vi "Measurement Logic.vi"() -> ()   [LabVIEW 2024, in "Averaged - Broadband.lvlib"]
uses:
  Averaged - Broadband.lvlib
  <vilib>/Plug-In SDKs/Measurements/Measure Call Context/Measure Call Context.lvclass
  Measurement Configuration.ctl
  Measurement Results.ctl
  <vilib>/addons/_NISVFA/_Generation/Signal Generation/SV Signal/sv_System Timing Model.ctl
  Program Files/NI/LVAddons/nisvt/1/examples/Sound and Vibration/Audio Measurements/subVIs/sv_AI Channel Configuration.ctl
  Program Files/NI/LVAddons/nisvt/1/examples/Sound and Vibration/Audio Measurements/subVIs/sv_AO Channel Configuration.ctl
  <vilib>/addons/_NISVFA/_Shared subVIs/Controls/NI Spectrum Component.ctl
  <vilib>/addons/_NISVFA/_Shared subVIs/Controls/svc_Window [Dual FFT].ctl
  <vilib>/addons/_NISVFA/_Generation/Signal Generation/SV Signal/SV Signal.lvclass/SV Signal.ctl
  <vilib>/addons/_NISVFA/_Generation/Signal Generation/SV Signal/Write Number of Averages.vi
  <extravilib>/ChannelInstances/High Speed Stream-a[.](wfm(dbl))/_Read For Replicate.vi
  <extravilib>/ChannelInstances/Tag-bool/Write.vi
  <vilib>/DAQmx/read.llb/DAQmx Read.vi
  <vilib>/DAQmx/read.llb/DAQmx Read (Analog 1D Wfm NChan NSamp Duration).vi
  <extravilib>/ChannelInstances/High Speed Stream-a[.](wfm(dbl))/Write.vi
  <vilib>/DAQmx/write.llb/DAQmx Write.vi
  <vilib>/DAQmx/write.llb/DAQmx Write (Analog Wfm 1Chan NSamp).vi
  Program Files/NI/LVAddons/nisvt/1/examples/Sound and Vibration/Audio Measurements/subVIs/sv_Synchronization Gatekeeper.vi
  <vilib>/Utility/error.llb/Clear Errors.vi
  Program Files/NI/LVAddons/nisvt/1/examples/Sound and Vibration/Audio Measurements/subVIs/sv_Align and Parse for Stimulus Response.vi
  Program Files/NI/LVAddons/nisvt/1/examples/Sound and Vibration/Audio Measurements/subVIs/sv_Synchronize Acquisition and Generation.vi
  Program Files/NI/LVAddons/nisvt/1/examples/Sound and Vibration/Audio Measurements/subVIs/sv_Synchronize DSA AI and AO Tasks.vi
  <extravilib>/ChannelInstances/Tag-bool/Read With Abort.vi
  <extravilib>/ChannelInstances/Tag-bool/Write With Abort.vi
  Program Files/NI/LVAddons/nisvt/1/examples/Sound and Vibration/Audio Measurements/subVIs/sv_Prepare Acquired Waveforms for Parsing.vi
  Program Files/NI/LVAddons/nisvt/1/examples/Sound and Vibration/Audio Measurements/subVIs/sv_Timing for Stimulus Response Tasks.vi
  <vilib>/addons/_NISVFA/_Generation/Signal Generation/SV Signal/Read Total Samples.vi
  <vilib>/addons/_NISVFA/_Generation/Signal Generation/SV Signal/Write Leading Synchronization Pulse Enable.vi
  Program Files/NI/LVAddons/nisvt/1/examples/Sound and Vibration/Audio Measurements/subVIs/sv_Synchronization Keymaster.vi
  Program Files/NI/LVAddons/nisvt/1/examples/Sound and Vibration/Audio Measurements/subVIs/sv_Get Reference Clock.vi
  Program Files/NI/LVAddons/nisvt/1/examples/Sound and Vibration/Audio Measurements/subVIs/sv_Synchronization Keymaster_GO.vi
  <extravilib>/ChannelInstances/Tag-c(ref(UserDefinedRefnumTag),t'Rendezvous RefNum')/Read With Abort.vi
  Program Files/NI/LVAddons/nisvt/1/examples/Sound and Vibration/Audio Measurements/subVIs/sv_Align Waveforms by Leading Sync Pulse.vi
  <vilib>/addons/_NISVFA/_Generation/Signal Generation/SV Signal/Read Synchronization Pulse Waveform.vi
  <vilib>/addons/_NISVFA/_Shared subVIs/Common/svc_Check for Waveform Parameter Continuity (N Ch).vi
  Program Files/NI/LVAddons/nisvt/1/examples/Sound and Vibration/Audio Measurements/subVIs/sv_Append Virtual Reference.vi
  <vilib>/addons/_NISVFA/_Generation/Signal Generation/SV Signal/Calculate Number of Remaining Samples.vi
  <extravilib>/ChannelInstances/Tag-c(ref(UserDefinedRefnumTag),t'Rendezvous RefNum')/Write.vi
  Program Files/NI/LVAddons/nisvt/1/examples/Sound and Vibration/Audio Measurements/subVIs/sv_Measure Delay for Active and Idle Channels.vi
  <vilib>/addons/_NISVFA/_Generation/Signal Generation/SV Signal/Read Leading Synchronization Pulse Enable.vi
  <vilib>/addons/_NISVFA/_Generation/Signal Generation/SV Signal/Read Trailing Synchronization Pulse Enable.vi
  <vilib>/addons/_NISVFA/_Shared subVIs/Common/svc_Check for Waveform Parameter Continuity (no state).vi
  <vilib>/addons/_NISVFA/_Shared subVIs/Common/sv_Get NI Property Name String.vi
  <extravilib>/ChannelInstances/Tag-c(ref(UserDefinedRefnumTag),t'Rendezvous RefNum')/Write With Abort.vi
  <vilib>/addons/Sound and Vibration/svt_Calibration/SV Measure Delay and Polarity and Coherence (Nx1).vi
  Program Files/NI/LVAddons/nisvt/1/examples/Sound and Vibration/Audio Measurements/subVIs/sv_Assign Delay to Idle Channels.vi
  <vilib>/addons/_NISVFA/_Shared subVIs/Common/svc_Get SV Channel Info.vi
  <vilib>/addons/Sound and Vibration/svt_Calibration/SV Measure Delay and Polarity and Coherence.vi
  <vilib>/addons/_NISVFA/_Shared subVIs/Common/svc_Unit Label to Engineering Units.vi
  <vilib>/addons/_NISVFA/_Shared subVIs/Common/svc_Engineering Units to Unit Label.vi
  <vilib>/Analysis/_algsub.llb/Vector Norm.vi
  <vilib>/Analysis/_algsub.llb/Real Vector Norm.vi
  <vilib>/addons/_NISVFA/_Shared subVIs/Common/SV Get Data Subset.vi
  <vilib>/addons/_NISVFA/_Shared subVIs/Common/svc_Get Array Subset (Index).vi
  <vilib>/addons/_NISVFA/_Shared subVIs/Common/svc_Coerce Index and Length.vi
  <vilib>/addons/_NISVFA/_Shared subVIs/Common/svc_Conditional Merge Error.vi
  <vilib>/addons/_NISVFA/_Generation/Signal Generation/SV Noise/SV Noise.lvclass
  C:/Program Files/NI/LVAddons/nisvt/1/vi.lib/addons/_NISVFA/_Generation/Signal Generation/SV Signal/SV Signal.lvclass
  <extravilib>/ChannelInstances/Tag-bool/Instantiate.vi
  <extravilib>/ChannelInstances/High Speed Stream-a[.](wfm(dbl))/Instantiate.vi
  <vilib>/addons/_NISVFA/_Generation/Signal Generation/SV Noise/Configure White Noise.vi
  <vilib>/addons/_NISVFA/_Generation/Signal Generation/SV Noise/Configure Pink Noise.vi
  <vilib>/addons/_NISVFA/_Generation/Signal Generation/SV Noise/Configure Periodic Random Noise.vi
  <vilib>/addons/_NISVFA/_Generation/Signal Generation/SV Signal/Write System Timing Model.vi
  <vilib>/addons/_NISVFA/_Generation/Signal Generation/SV Signal/Write Measurement Duration.vi
  <vilib>/addons/_NISVFA/_Generation/Signal Generation/SV Signal/Write Pre-Measurement Settling Duration.vi
  <vilib>/addons/_NISVFA/_Generation/Signal Generation/SV Signal/Write Minimum Value.vi
  <vilib>/addons/_NISVFA/_Generation/Signal Generation/SV Signal/Write Maximum Value.vi
  <vilib>/addons/_NISVFA/_Generation/Signal Generation/SV Signal/Write Transition Profile.vi
  <vilib>/addons/_NISVFA/_Generation/Signal Generation/SV Signal/Write Ramp Parameters.vi
  <extravilib>/ChannelInstances/High Speed Stream-a[.](wfm(dbl))/)Channel.vi
  <extravilib>/ChannelInstances/High Speed Stream-a[.](wfm(dbl))/Abort Signal/Init Signal.vi
  <vilib>/addons/_NISVFA/_Baseband FFT/SVFA Frequency Response (1x1) (Mag-Phase).vi
  <extravilib>/ChannelInstances/Tag-bool/EndpointRead.vi
  <extravilib>/ChannelInstances/Tag-bool/Endpoint.vi
  <extravilib>/ChannelInstances/Tag-c(ref(UserDefinedRefnumTag),t'Rendezvous RefNum')/Instantiate.vi
  Program Files/NI/LVAddons/nisvt/1/examples/Sound and Vibration/Audio Measurements/subVIs/sv_Configure AI Task.vi
  Program Files/NI/LVAddons/nisvt/1/examples/Sound and Vibration/Audio Measurements/subVIs/sv_Configure AO Task.vi
  <vilib>/addons/_NISVFA/_Generation/Signal Generation/SV Signal/Read Sample Rate.vi
  <vilib>/addons/_NISVFA/_Generation/Signal Generation/SV Signal/Read Generation State.vi
  <vilib>/addons/_NISVFA/_Generation/Signal Generation/SV Signal/Read System Timing Model.vi
  <vilib>/DAQmx/configure/timing.llb/DAQmx Timing.vi
  <vilib>/DAQmx/configure/timing.llb/DAQmx Timing (Sample Clock).vi
  <vilib>/addons/_NISVFA/_Generation/Signal Generation/SV Signal/Write Sample Rate.vi
  <vilib>/DAQmx/configure/task.llb/DAQmx Stop Task.vi
  Program Files/NI/LVAddons/nisvt/1/examples/Sound and Vibration/Audio Measurements/subVIs/sv_Get Bus Type and Product Type.vi
  <vilib>/DAQmx/configure/task.llb/DAQmx Control Task.vi
  <vilib>/Utility/rendezvs.llb/Create Rendezvous.vi
  <vilib>/Utility/rendezvs.llb/Wait at Rendezvous.vi
  <extravilib>/ChannelInstances/Tag-c(ref(UserDefinedRefnumTag),t'Rendezvous RefNum')/Endpoint.vi
  <vilib>/addons/Sound and Vibration/svt_DAQmx/subVIs/svl_Get Terminal Name with Device Prefix.vi
  <vilib>/DAQmx/configure/trigger.llb/DAQmx Trigger.vi
  <vilib>/DAQmx/configure/trigger.llb/DAQmx Start Trigger (Digital Edge).vi
  <vilib>/DAQmx/configure/task.llb/DAQmx Start Task.vi
  <extravilib>/ChannelInstances/Tag-c(ref(UserDefinedRefnumTag),t'Rendezvous RefNum')/EndpointRead.vi
  <vilib>/Utility/rendezvs.llb/Destroy Rendezvous.vi
  <vilib>/DAQmx/miscellaneous.llb/DAQmx Fill In Error Info.vi
  <vilib>/DAQmx/configure/task.llb/DAQmx Clear Task.vi
  <vilib>/Utility/LVClass/Get LV Class Name.vi
  <vilib>/addons/_NISVFA/_Shared subVIs/Data Objects/Waveforms (DBL)/Write to Buffer.vi
  <vilib>/addons/_NISVFA/_Shared subVIs/Data Objects/Waveforms (DBL)/Read from Buffer.vi
  <vilib>/addons/_NISVFA/_Shared subVIs/Data Objects/Waveforms (DBL)/SV Read Newest Data.vi
  <vilib>/measure/maresamp.llb/Resample Waveforms (single shot).vi
  <vilib>/measure/maresamp.llb/Resample Waveform (single shot).vi
  <vilib>/addons/_NISVFA/_Shared subVIs/Common/svc_Check dt for Equal Sample Rates.vi
  <vilib>/Waveform/TSOps.llb/Timestamp Subtract.vi
  <vilib>/Analysis/2dsp.llb/CrossCorrelation.vi
  <vilib>/Analysis/2dsp.llb/1D Cross Correlation (DBL).vi
  <vilib>/addons/_NISVFA/_Shared subVIs/Common/svc_Fit Quadratic to Max Three Points in Array.vi
  <vilib>/Utility/error.llb/Error Cluster From Error Code.vi
  <vilib>/addons/_NISVFA/_Shared subVIs/Common/svc_Caller VI Returned in Error Source.vi
  <vilib>/addons/_NISVFA/_Shared subVIs/Common/SV Remove Delays (1,N) from Waveforms (N Ch) (DBL).vi
  <vilib>/addons/_NISVFA/_Shared subVIs/Common/SV Remove Delays from Waveforms.vi
  <vilib>/addons/_NISVFA/_Shared subVIs/Data Objects/Waveforms (DBL)/SV Read Next Measurement Data.vi
  <vilib>/DAQmx/configure/task.llb/DAQmx Wait Until Done.vi
  <extravilib>/ChannelInstances/Event Messenger-bool/Instantiate.vi
  <vilib>/addons/_NISVFA/_Generation/Signal Generation/SV Signal/SV Signal.lvclass
  <vilib>/addons/_NIFileIO/SV TDMS Write Spectrum (1 Ch).vi
  <extravilib>/ChannelInstances/High Speed Stream-a[.](wfm(dbl)).lvlib
  Program Files/NI/LVAddons/nisvt/1/examples/Sound and Vibration/SoundVib_Audio Examples.lvlib
  aa5de61b-977d-4362-be53-9449d164fb1b.vi
panel:
  in  "stop":bool
  out "measurement results":T1={"averages completed"=0.0, "f0"=0.0, "df"=0.0, "coherence"=[0.0], "magnitude"=[0.0], "phase"=[0.0], "FRF file path"="Empty"}
  in  "measurement configuration":T2={"sample rate"=1.2, "ao stimulus channel"="Lorem ipsum dolor sit", "ao range"=32.0, "ao terminal configuration"=32, "ai reference channel"="Dev1/ai0", "ai ref range"=64.0, "ai reference terminal configuration"=-32, "ai response channel"="Dev1/ai1", "ai response range"=-64.0, "ai response terminal configuration"=-64, "level"=1.0, "frequency resolution"=1.0, "averages"=1, "signal type"=1, "averaging mode"=2} {"averaging mode" items=["No averaging", "Vector averaging", "RMS averaging", "Peak hold"]; "signal type" items=["Rabbit", "Gopher", "Badger"]; "frequency resolution" format="%#_4f Hz"; "level" format="%#_6f Vrms"; "ai response range" format="± %#_6f V"; "ao range" format="± %#_4f V"; "sample rate" format="%#.2p Hz"}
  out "measure call context out":refnum<class "Measure Call Context.lvclass">
  in  "measure call context in":refnum<class "Measure Call Context.lvclass">
  out "error out":errorcluster
  in  "error in":errorcluster
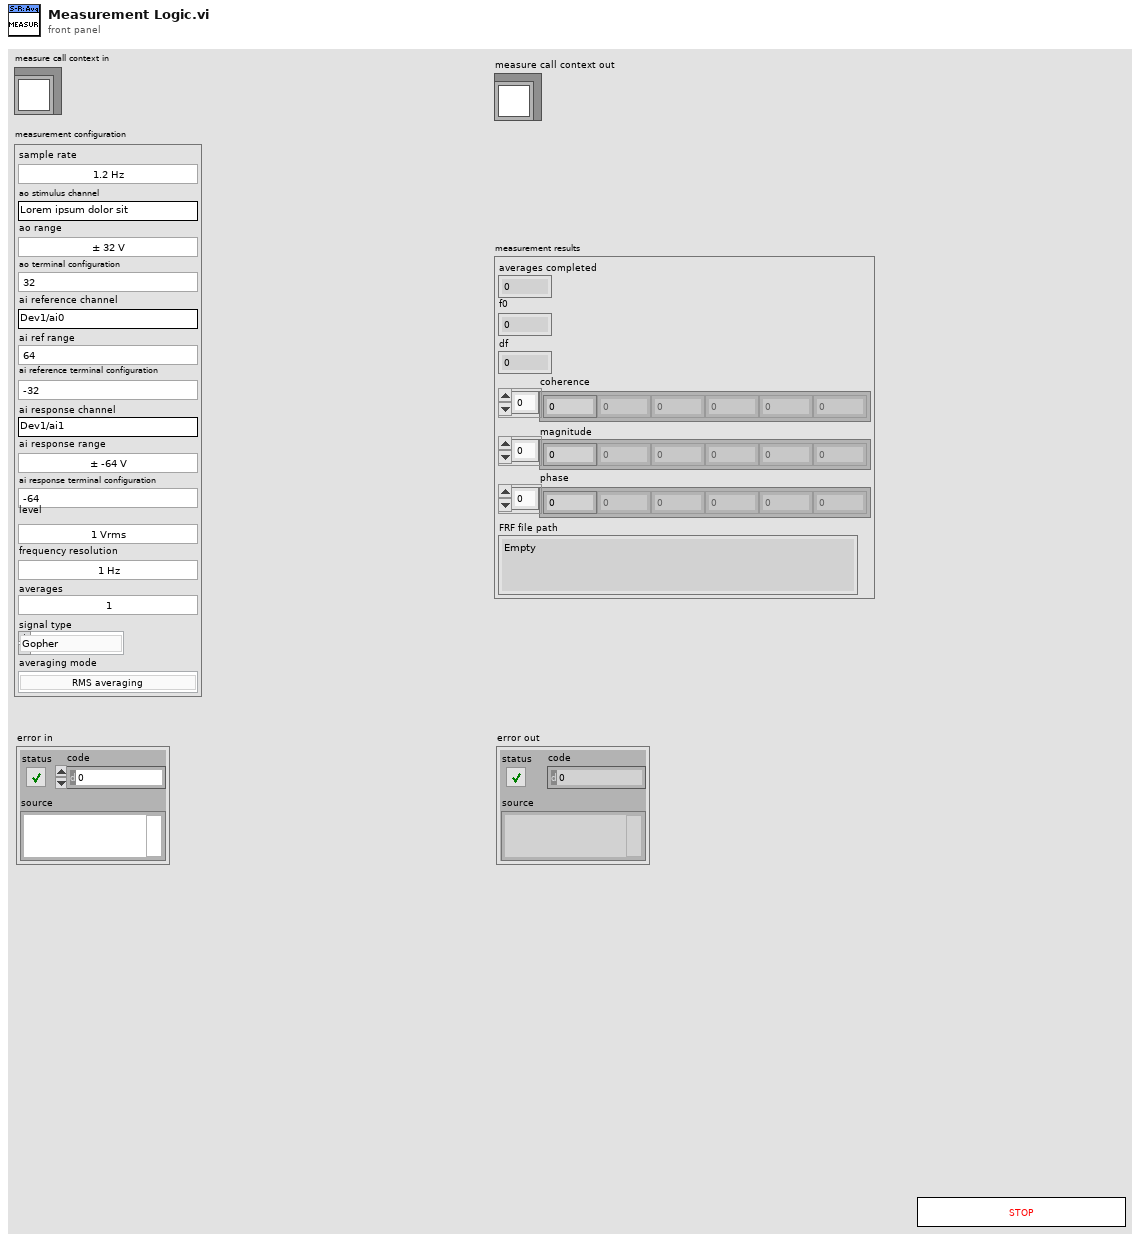
[diagram p1: front panel]
types:
  T1 = typedef "Averaged - Broadband.lvlib/Measurement Results.ctl" = cluster{"averages completed":dbl, "f0":dbl, "df":dbl, "coherence":dbl[], "magnitude":dbl[], "phase":dbl[], "FRF file path":string}
  T2 = typedef "Averaged - Broadband.lvlib/Measurement Configuration.ctl" = cluster{"sample rate":dbl, "ao stimulus channel":string, "ao range":dbl, "ao terminal configuration":i32, "ai reference channel":string, "ai ref range":dbl, "ai reference terminal configuration":i32, "ai response channel":string, "ai response range":dbl, "ai response terminal configuration":i32, "level":dbl, "frequency resolution":dbl, "averages":i32, "signal type":i32, "averaging mode":i32}
  T3 = enum16{"Uniform white noise", "Gaussian white noise", "Pink noise", "Periodic random noise"}
  T4 = enum16{"open", "open or create", "create or replace", "create", "open (read-only)"}
  T5 = cluster{"averaging mode":enum16{"No averaging", "Vector averaging", "RMS averaging", "Peak hold"}, "weighting mode":enum16{"Linear", "Exponential"}, "number of averages":u32, "linear mode":enum16{"One shot", "Auto restart"}}
  T6 = typedef "SoundVib_Audio Examples.lvlib/sv_AO Channel Configuration.ctl" = cluster{"DAQmx Channel":tag, "Max":dbl, "output terminal configuration":i32}
  T7 = cluster{"profile":enum16{"Linear", "Half cosine"}, "durations [s]":cluster{"ramp-up":dbl, "transition":dbl, "ramp-down":dbl}}
  T8 = typedef "NI Spectrum Component.ctl" = u16
  T9 = typedef "SoundVib_Audio Examples.lvlib/sv_AI Channel Configuration.ctl" = cluster{"DAQmx Channel":tag, "Channel Type":u16, "Max":dbl, "Sensitivity":dbl, "Coupling":enum16{"AC", "DC"}, "excitation":enum16{"Off", "Min", "Max"}, "input terminal configuration":i32}
  T10 = typedef "SV Signal.lvclass/sv_System Timing Model.ctl" = i64
  T11 = typedef "High Speed Stream-a[.](wfm(dbl)).lvlib/)Channel.ctl" = refnum<queue>
  T12 = typedef "svc_Window [Dual FFT].ctl" = u32
  T13 = typedef "svc_Spectrum Info.ctl" = cluster{"channel name":string, "description":string, "x-axis units":T14, "spectral info":cluster{"spectrum type":T15, "linear/dB":enum16{"linear", "dB"}, "window":u16, "window size":i32, "FFT size":i32}, "engineering units":T16, "custom label":string, "dB reference [EU]":dbl, "peak units":enum16{"rms", "peak", "peak-peak"}, "weighting filter":T17, "spectral density?":bool, "unit label":string, "spectrum skewed?":bool, "complimentary spectrum units":T18}
  T14 = typedef "svc_X-Axis Units.ctl" = u16
  T15 = typedef "svc_Spectrum Type.ctl" = enum16{"FFT Spectrum [complex]", "Amplitude [Magnitude]", "Power [Magnitude^2]", "Cross Spectrum [complex]", "Frequency Response [Complex]"}
  T16 = typedef "svc_Engineering Units Text Ring.ctl" = u16
  T17 = typedef "svc_Weighting Filter Text Ring.ctl" = u16
  T18 = typedef "svc_Complimentary Spectrum Units.ctl" = enum16{"none", "radians", "degrees", "cycles", "imaginary"}
  T19 = typedef "Event Messenger-bool.lvlib/))Channel.ctl" = refnum<queue>
  T20 = typedef "Tag-bool.lvlib/))Channel.ctl" = refnum<queue>
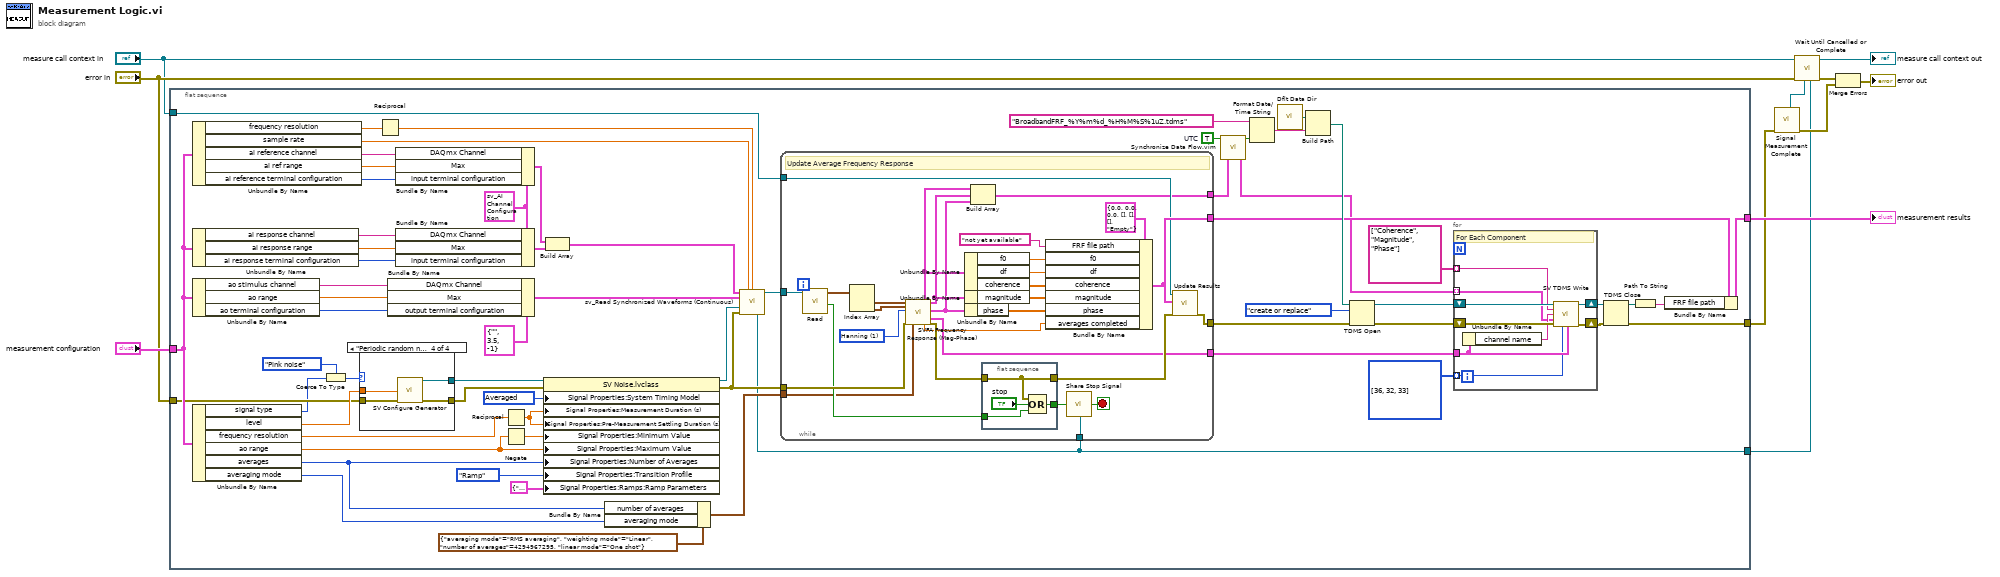
[diagram p0: block diagram]
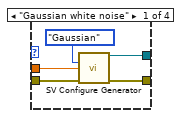
[diagram p2: hidden frame]
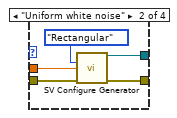
[diagram p3: hidden frame]
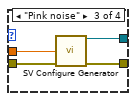
[diagram p4: hidden frame]
diagram:
  n1 = flat-sequence {
    tunnel: "measurement configuration" -> [w40]
    tunnel: [w24] -> w10
    tunnel: "error in" -> [w39]
    tunnel: [w27] -> w7
    tunnel: w2 -> [w44]
    tunnel: "measure call context in" -> [w32]
    frame #0 {
      w16 = T8[] [36, 32, 33] items=["Magnitude^2"=37, "Magnitude"=32, "Phase"=33, "Real"=34, "Imaginary"=35, "Coherence"=36, "Unknown"=99]
      w15 = TRUE  # UTC
      w69 = T9 {"DAQmx Channel"="", "Channel Type"=0, "Max"=3.0, "Sensitivity"=1000.0, "Coupling"=enum."DC", "excitation"=enum."Off", "input terminal configuration"=-1} ("Channel Information")
      w38 = T10 210123 items=["Finite"=10178, "-"=-1, "Continuous"=10123, "-"=-2, "Settled"=110123, "Averaged"=210123, "Discrete Sweep"=310123, "Continuous Sweep"=410123] ("System Timing Model")
      n2 = Unbundle By Name(w40) -> ("frequency resolution"=w57:dbl, "sample rate"=w58:dbl, "ai reference channel"=w61:string, "ai ref range"=w60:dbl, "ai reference terminal configuration"=w59:i32)
      n3 = Unbundle By Name(w40) -> ("ai response channel"=w43:string, "ai response range"=w42:dbl, "ai response terminal configuration"=w41:i32)
      n4 = Unbundle By Name(w40) -> ("ao stimulus channel"=w55:string, "ao range"=w54:dbl, "ao terminal configuration"=w53:i32)
      n5 = Unbundle By Name(w40) -> ("signal type"=w22:i32, "level"=w52:dbl, "frequency resolution"=w50:dbl, "ao range"=w51:dbl, "averages"=w45:i32, "averaging mode"=w48:i32)
      n6 = Coerce To Type(0:w22, 1:T3."Pink noise" ("signal type")) -> (2:w21:T3)
      n7 = case shown="\"Periodic random noise\"" w21 {
        tunnel: [w89 w94 w98 w102] -> w75
        tunnel: [w88 w93 w97 w101] -> w63
        tunnel: w52 -> [w87 w92 w96 w100]
        tunnel: w39 -> [w85 w90 w95 w99]
        frame "Gaussian white noise" {
          n8 = call-poly <vilib>:"SV Configure Generator.vi"("amplitude PDF"=enum16{"Gaussian", "Rectangular", "Triangular"}."Gaussian", "level"=w87, "error in (no error)"=w85) -> ("signal configuration"=w89:refnum<class "SV Noise.lvclass">, "error out"=w88:errorcluster)  [unwired: 11 in]
        }
        frame "Uniform white noise" {
          n9 = call-poly <vilib>:"SV Configure Generator.vi"("amplitude PDF"=enum16{"Gaussian", "Rectangular", "Triangular"}."Rectangular", "level"=w92, "error in (no error)"=w90) -> ("signal configuration"=w94:refnum<class "SV Noise.lvclass">, "error out"=w93:errorcluster)  [unwired: 11 in]
        }
        frame "Pink noise" {
          n10 = call-poly <vilib>:"SV Configure Generator.vi"("level"=w96, "error in"=w95) -> ("signal configuration"=w98:refnum<class "SV Noise.lvclass">, "error out"=w97:errorcluster)  [unwired: 12 in]
        }
        frame "Periodic random noise" {
          n11 = call-poly <vilib>:"SV Configure Generator.vi"("level"=w100, "error in (no error)"=w99) -> ("signal configuration"=w102:refnum<class "SV Noise.lvclass">, "error out"=w101:errorcluster)  [unwired: 12 in]
        }
      }
      n12 = Reciprocal(x=w57) -> (1/x=w56:dbl)
      n13 = Bundle By Name(cluster=T6 {"DAQmx Channel"="", "Max"=3.5, "output terminal configuration"=-1} ("analog output channel"), "DAQmx Channel"=w55, "Max"=w54, "output terminal configuration"=w53) -> (w64:T6)
      n14 = Bundle By Name(cluster=w69, "DAQmx Channel"=w61, "Max"=w60, "input terminal configuration"=w59) -> (w67:T9)
      n15 = Bundle By Name(cluster=w69, "DAQmx Channel"=w43, "Max"=w42, "input terminal configuration"=w41) -> (w66:T9)
      n16 = Reciprocal(x=w50) -> (1/x=w46:dbl)
      n17 = Negate(x=w51) -> (-x=w62:dbl)
      n18 = property class="SV Noise.lvclass"(reference=w75, error in=w63, "Signal Properties:System Timing Model"=w38, "Signal Properties:Measurement Duration (s)"=w46, "Signal Properties:Pre-Measurement Settling Duration (s)"=w46, "Signal Properties:Minimum Value"=w62, "Signal Properties:Maximum Value"=w51, "Signal Properties:Number of Averages"=w45, "Signal Properties:Transition Profile"=enum16{"Immediate", "Next optimum", "Ramp"}."Ramp" ("Transition Profile"), "Signal Properties:Ramps:Ramp Parameters"=T7 {"profile"=enum."Half cosine", "durations [s]"={"ramp-up"=0.1, "transition"=0.0, "ramp-down"=0.1}} ("Ramp Parameters")) -> (reference out=w70:refnum<class "SV Noise.lvclass">, error out=w71:errorcluster)
      n19 = Build Array(w67, w66) -> (w65:T9[])
      n20 = Bundle By Name(cluster=T5 {"averaging mode"=enum."RMS averaging", "weighting mode"=enum."Linear", "number of averages"=4294967295, "linear mode"=enum."One shot"} ("averaging parameters"), "number of averages"=w45, "averaging mode"=w48) -> (w47:T5)
      n21 = call "sv_Read Synchronized Waveforms (Continuous).vi"("ai channels"=w65, "sample rate (Hz)"=w58, "block duration (s)"=w56, "ao channel"=w64, "signal configuration"=w70, "error in"=w71, "stop channel"=w44) -> ("measurement channel"=w72:T11)  [unwired: 7 in, 1 out]
      n22 = while {
        tunnel: w71 -> [w127]
        tunnel: w72 -> [w124]
        tunnel: w44 -> [w123]
        tunnel: w47 -> [w122]
        tunnel: [w120] -> w28
        tunnel: [w117] -> w26
        tunnel: w32 -> [w116]
        tunnel: [w107] -> w20
        tunnel: [w103] -> w13
        stop <- w130 stop-if-true
        w128 = T12 1 items=["None"=0, "Hanning"=1, "Hamming"=2, "Blackman-Harris"=3, "Exact Blackman"=4, "Blackman"=5, "Flat Top"=6, "4 Term B-Harris "=7, "7 Term B-Harris"=8, "Low Sidelobe"=9, "Force - Exponential"=10, "Force"=64, "Exponential"=65, "Blackman Nuttall"=11, "Triangle"=30, "Bartlett-Hanning"=31, "Bohman"=32, "Parzen"=33, "Welch"=34, "Kaiser"=60, "Dolph-Chebyshev"=61, "Gaussian"=62] ("window")
        # "Update Average Frequency Response"
        n23 = call <extravilib>:"Read.vi"("channel"=w124) -> ("done?"=w126:bool, "element"=w114:waveform(dbl)[])  [unwired: 6 in, 3 out]
        n24 = Index Array(array=w114) -> (element #1=w125:waveform(dbl), element #2=w113:waveform(dbl))  [unwired: 2 in]
        n25 = call-poly <vilib>:"SVFA Frequency Response (Mag-Phase).vi"("stimulus signal X [EUx]"=w125, "response signal Y [EUy]"=w113, "window"=w128, "error in (no error)"=w127, "averaging parameters"=w122) -> ("coherence"=w106:cluster{"f0":dbl, "df":dbl, "coherence":dbl[]}, "averages completed"=w118:dbl, "magnitude [dB EUy/EUx]"=w105:cluster{"f0":dbl, "df":dbl, "magnitude":dbl[]}, "phase [degrees]"=w104:cluster{"f0":dbl, "df":dbl, "phase":dbl[]}, "spectrum info"=w107:T13, "error out"=w129:errorcluster)  [unwired: 6 in, 3 out]
        n26 = Unbundle By Name(w106) -> ("f0"=w112:dbl, "df"=w111:dbl, "coherence"=w110:dbl[])
        n27 = Unbundle By Name(w105) -> ("magnitude"=w109:dbl[])
        n28 = Unbundle By Name(w104) -> ("phase"=w108:dbl[])
        n29 = Build Array(w106, w105, w104) -> (w103:cluster{"f0":dbl, "df":dbl, "phase":dbl[]}[])
        n30 = flat-sequence {
          tunnel: w126 -> [w135]
          tunnel: [w133] -> w131
          tunnel: w129 -> [w132]
          tunnel: [w132] -> w121
          frame #0 {
            n31 = Compound Arithmetic op=OR(w132, "stop", w135) -> (w133:bool)
          }
        }
        n32 = Bundle By Name(cluster=T1 {"averages completed"=0.0, "f0"=0.0, "df"=0.0, "coherence"=[], "magnitude"=[], "phase"=[], "FRF file path"="Empty"} ("Measurement Results"), "FRF file path"="not yet available", "f0"=w112, "df"=w111, "coherence"=w110, "magnitude"=w109, "phase"=w108, "averages completed"=w118) -> (w117:T1)
        n33 = call <vilib>:"Share Stop Signal.vi"("set stop (F)"=w131, "channel"=w123) -> ("stop"=w130:bool)
        n34 = call <vilib>:"Update Results.vi"("error in"=w121, "measurement results"=w117, "measure call context in"=w116) -> ("error out"=w120:errorcluster)  [unwired: 7 in, 1 out]
      }
      n35 = call "Synchronize Data Flow.vim"("input 4"=w13, "input 1"=w15) -> ("output 4"=w12:cluster{"f0":dbl, "df":dbl, "phase":dbl[]}[], "output 1"=w14:bool)  [unwired: 2 in, 2 out]
      n36 = Format Date/Time String(time format string (%c)="BroadbandFRF_%Y%m%d_%H%M%S%1uZ.tdms", UTC format=w14) -> (date/time string=w34:string)  [unwired: 1 in]
      n37 = call <vilib>:"Dflt Data Dir.vi"() -> ("App:Default Data Directory"=w35:path)
      n38 = Build Path(base path=w35, name or relative path=w34) -> (appended path=w33:path)
      n39 = TDMS Open(8:w28, 10:T4."create or replace" ("operation (0:open)"), 11:w33) -> (0:w29:errorcluster, 3:w30:refnum<k34>)  [unwired: 4 in]
      n40 = for {
        tunnel: w20 -> [w82]
        shift-right: [w80] -> w18
        shift-left: w30 -> [w84]
        shift-right: [w79] -> w19
        shift-left: w29 -> [w83]
        tunnel: string[] ["Coherence", "Magnitude", "Phase"] -> [w78] mode=indexing
        tunnel: w16 -> [w77] mode=indexing
        tunnel: w12 -> [w76] mode=indexing
        # "For Each Component"
        n41 = Unbundle By Name(w82) -> ("channel name"=w81:string)
        n42 = call-poly <vilib>:"SV TDMS Write.vi"("tdms file"=w84, "group name in"=w78, "channel name in"=w81, "spectrum"=w76, "error in"=w83, "component"=w77, "spectrum info"=w82) -> ("tdms file out"=w80:refnum<k34>, "error out"=w79:errorcluster)  [unwired: 5 in, 2 out]
      }
      n43 = TDMS Close(8:w19, 11:w18) -> (0:w27:errorcluster, 3:w31:path)
      n44 = Path To String(path=w31) -> (string=w25:string)
      n45 = Bundle By Name(cluster=w26, "FRF file path"=w25) -> (w24:T1)
    }
  }
  n46 = call "Signal Measurement Complete.vi"("error in (no error)"=w7) -> ("error out"=w5:errorcluster, "done channel"=w6:T19)  [unwired: 9 in]
  n47 = call "Wait Until Cancelled or Complete.vi"("done channel"=w6, "error in (no error)"="error in", "measure call context in"="measure call context in") -> ("error out"=w4:errorcluster, "measure call context out"=→"measure call context out":refnum<class "Measure Call Context.lvclass">, "channel"=w2:T20)  [unwired: 6 in]
  n48 = Merge Errors(w4, w5) -> (→"error out":errorcluster)
  "measurement results" <- w10
